vi "DigitalLed.vi"() -> ()   [LabVIEW 2015]
panel:
  out "LED 2":bool[](array[boolean])
  out "LED 1":bool[](array[boolean])
  in  "stop":bool
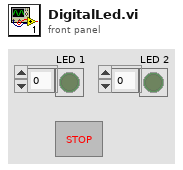
[diagram p1: front panel]
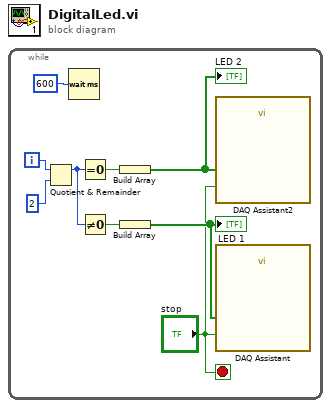
[diagram p0: block diagram]
diagram:
  n1 = while {
    i -> [w9]
    stop <- "stop" stop-if-true
    n2 = Quotient & Remainder(x=w9, y=2) -> (x-y*floor(x/y)=w5:i32)  [unwired: 1 out]
    n3 = Wait (ms)(milliseconds to wait=u32 600) -> ()  [unwired: 1 out]
    n4 = Equal To 0?(x=w5) -> (x = 0?=w3:bool)
    n5 = Not Equal To 0?(x=w5) -> (x != 0?=w4:bool)
    n6 = Build Array "Build Array"(w3) -> (w2:bool[])
    "LED 2" <- w2
    n7 = Build Array "Build Array"(w4) -> (w6:bool[])
    "LED 1" <- w6
    n8 = call "DAQ Assistant2"("data"=w2, "stop (T)"="stop") -> ()  [unwired: 16 in, 2 out]
    n9 = call "DAQ Assistant"("data"=w6, "stop (T)"="stop") -> ()  [unwired: 16 in, 2 out]
  }
